vi "ConfigOutputEnable.vi"(8 "error in (no error)":errorcluster, 11 "ClassIn":refnum<class "Keysight335XX.lvclass">) -> (0 "error out":errorcluster, 3 "ClassOut":refnum<class "Keysight335XX.lvclass">)   [LabVIEW 2014, in "FGenPlugins.lvlib" / "Keysight335XX.lvclass"]
uses:
  Keysight335XX.lvclass
  <instrlib>/Agilent 3352X Series/Agilent 3352X Series.lvlib
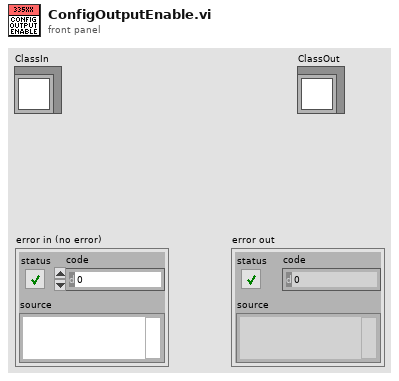
[diagram p1: front panel]
types:
  T1 = typedef "FGenPlugins.lvlib/NISTFGenPluginsBase.lvclass/ChannelParamElement.ctl" = cluster{"sName":string, "eOperateMode":u16, "bEnabled":bool, "eOutputMode":u16, "iIndex":i32, "iNameBufferSize":i32, "fGain":dbl}
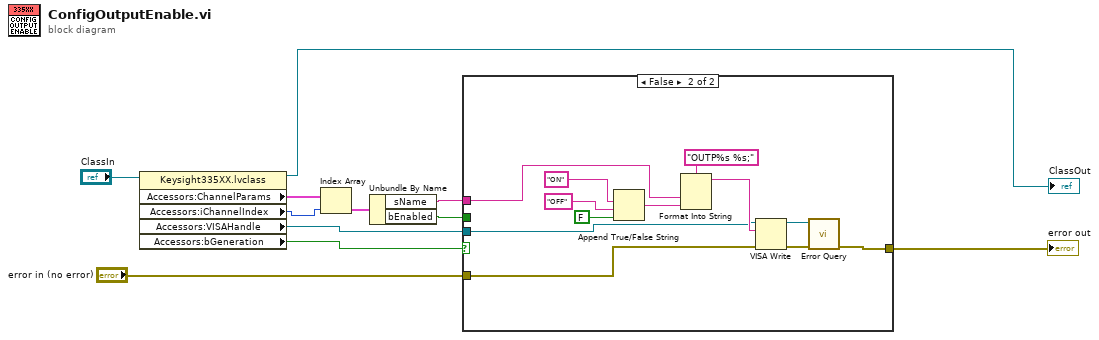
[diagram p0: block diagram]
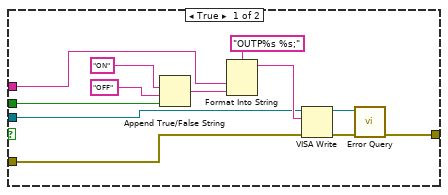
[diagram p2: hidden frame]
diagram:
  n1 = property class="Keysight335XX.lvclass"(reference="ClassIn") -> (reference out=→"ClassOut":refnum<class "Keysight335XX.lvclass">, "Accessors:ChannelParams"=w9:T1[], "Accessors:iChannelIndex"=w7:i32, "Accessors:VISAHandle"=w4:refnum<visa-resource-name>, "Accessors:bGeneration"=w2:bool)  [unwired: 1 in, 1 out]
  n2 = Index Array(array=w9, index=w7) -> (element=w8:T1)
  n3 = Unbundle By Name(w8) -> ("sName"=w5:string, "bEnabled"=w6:bool)
  n4 = case shown="False" w2 {
    tunnel: [w16 w28] -> w11
    tunnel: w6 -> [w15 _]
    tunnel: w5 -> [w14 w27]
    tunnel: w4 -> [w13 w26]
    tunnel: "error in (no error)" -> [w12 w25]
    frame True {
      n5 = Append True/False String(1:w15, 2:"OFF", 3:"ON") -> (0:w17:string)  [unwired: 1 out]
      n6 = Format Into String(format string="OUTP%s %s;", w14, w17) -> (resulting string=w19:string)  [unwired: 2 in, 1 out]
      n7 = VISA Write(VISA resource name=w13, write buffer=w19, error in (no error)=w12) -> (VISA resource name out=w20:refnum<visa-resource-name>, error out=w21:errorcluster)  [unwired: 1 out]
      n8 = call <instrlib>:"Error Query.vi"("error in (no error)"=w21, "VISA resource name"=w20) -> ("error out"=w16:errorcluster)  [unwired: 9 out]
    }
    frame False {
      n9 = Append True/False String(1:FALSE ("selector"), 2:"OFF", 3:"ON") -> (0:w29:string)  [unwired: 1 out]
      n10 = Format Into String(format string="OUTP%s %s;", w27, w29) -> (resulting string=w31:string)  [unwired: 2 in, 1 out]
      n11 = VISA Write(VISA resource name=w26, write buffer=w31, error in (no error)=w25) -> (VISA resource name out=w32:refnum<visa-resource-name>, error out=w33:errorcluster)  [unwired: 1 out]
      n12 = call <instrlib>:"Error Query.vi"("error in (no error)"=w33, "VISA resource name"=w32) -> ("error out"=w28:errorcluster)  [unwired: 9 out]
    }
  }
  "error out" <- w11
